vi "getAll.vi"(8 "error in (no error)":errorcluster, 11 "Sequence Experiment":refnum<class "Sequence Experiment.lvclass">) -> (0 "error out":errorcluster, 2 "getAll":variant, 3 "Sequence Experiment out":refnum<class "Sequence Experiment.lvclass">)   [LabVIEW 2016, in "Sequence Experiment.lvclass"]
uses:
  Sequence Experiment.lvclass
  <userlib>/LevyLab/Levylab Instruments/SMOs/Instrument/Instrument.lvclass
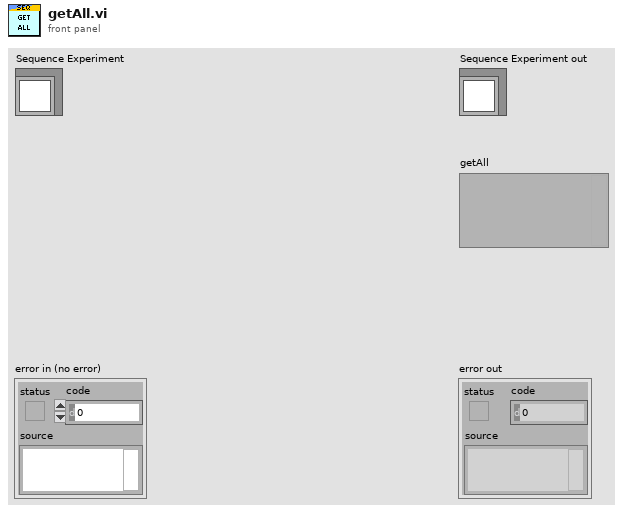
[diagram p1: front panel]
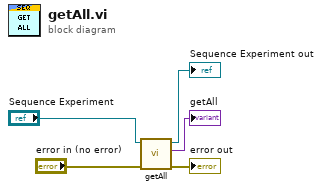
[diagram p0: block diagram]
diagram:
  n1 = call-parent "getAll.vi"("error in (no error)"="error in (no error)", "Instrument in"="Sequence Experiment") -> ("error out"=→"error out":errorcluster, "getAll"=→"getAll":variant, "Instrument out"=→"Sequence Experiment out":refnum<class "Sequence Experiment.lvclass">)  [unwired: 7 in]
